vi "MListbox Set Column Wide.vi"(8 "error in (no error)":errorcluster caption="错误输入（无错误）", 11 "Multicolumn ListBox 输入":refnum<class "Multicolumn ListBox.lvclass">) -> (0 "error out":errorcluster caption="错误输出", 3 "Multicolumn ListBox 输出":refnum<class "Multicolumn ListBox.lvclass">)   [LabVIEW 2018]
uses:
  Multicolumn ListBox.lvclass
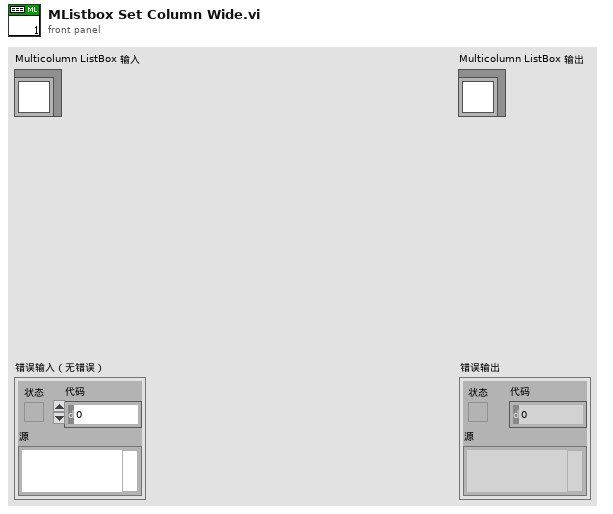
[diagram p1: front panel]
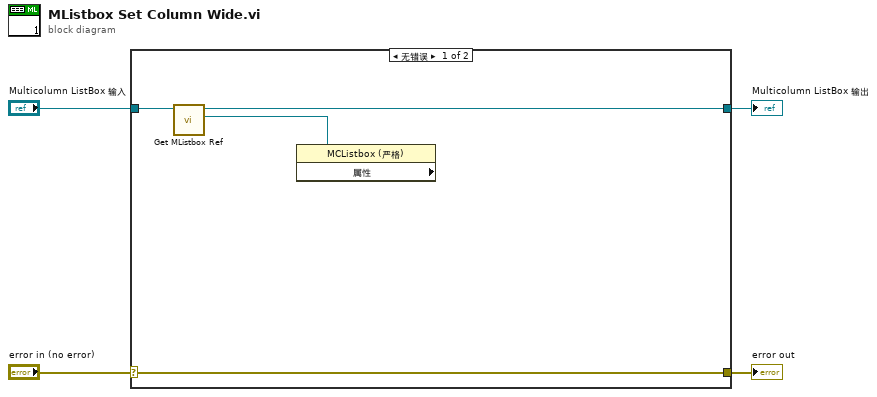
[diagram p0: block diagram]
diagram:
  n1 = case shown="无错误" "error in (no error)" {
    selector: "error in (no error)" -> [w8 w10]
    tunnel: [w8 w10] -> w3
    tunnel: [w6 w9] -> w1
    tunnel: "Multicolumn ListBox 输入" -> [w7 w9]
    frame No Error {
      n2 = call "Get MListbox Ref.vi"("Multicolumn ListBox in"=w7) -> ("MListbox Ref"=w5:refnum<vi>, "Multicolumn ListBox out"=w6:refnum<class "Multicolumn ListBox.lvclass">)  [unwired: 8 in, 1 out]
      n3 = property class="MCListbox (严格)" props=[](reference=w5) -> ()  [unwired: 1 in, 3 out]
    }
    frame Error {
    }
  }
  "error out" <- w3
  "Multicolumn ListBox 输出" <- w1
